vi "PH_GetSwitchInformation.contents.vi"   [LabVIEW 2014, in "PH_GetSwitchInformation.lvlib"]
doc: "This class is forseen to get information available in the PCS by reading the data base and alle nodes within the system.\n\nThis class is part of the PHELIX user layer."
uses:
  PH_GetSwitchInformation.lvlib
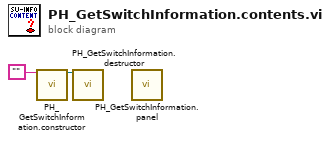
[diagram p0: block diagram]
diagram:
  n1 = call "PH_GetSwitchInformation.constructor.vi"("name"="") -> ("i ref out"=w1:refnum<vi>)  [unwired: 16 in, 2 out]
  n2 = call "PH_GetSwitchInformation.destructor.vi"("i ref in"=w1) -> ()  [unwired: 18 in, 1 out]
  n3 = call "PH_GetSwitchInformation.panel.vi"() -> ()  [unwired: 19 in, 1 out]
